vi "VdAnalogInput_Create.vi"(8 "Error In":errorcluster, 9 "VoltageRangeLow":dbl, 10 "VoltageRangeHigh":dbl, 11 "reference in":refnum<class "VdAnalogInput.lvclass">) -> (0 "Error Out":errorcluster, 3 "reference out":refnum<class "VdAnalogInput.lvclass">)   [LabVIEW 2020, in "VdAnalogInput.lvclass"]
uses:
  VdAnalogInput.lvclass
  VdAnalogInput.lvclass/VdAnalogInput.ctl
  VdInstrument_class/VdInstrument.lvclass
  C:/Projects/DesignPatterns/Factory1/VdInstrument_class/VdInstrument.lvclass
  C:/Projects/DesignPatterns/Factory1/VdAnalogInput_class/VdAnalogInput.lvclass
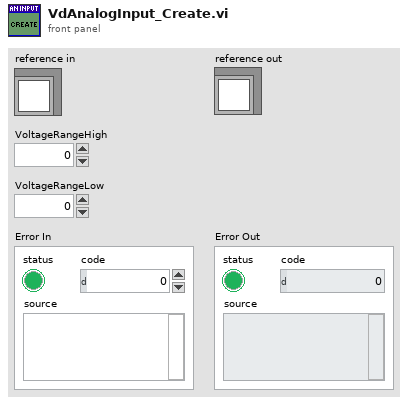
[diagram p1: front panel]
types:
  T1 = typedef "VdAnalogInput.lvclass/ObjectAttributes.ctl" = cluster{"LastReadValue":dbl, "VoltageRangeLow":dbl, "VoltageRangeHigh":dbl}
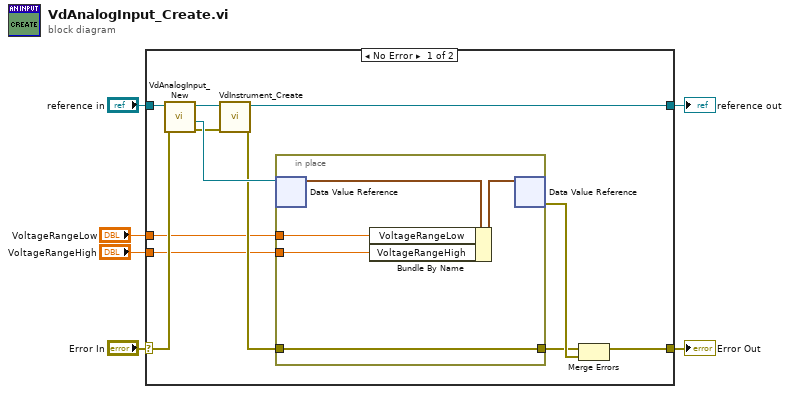
[diagram p0: block diagram]
diagram:
  n1 = case shown="No Error" "Error In" {
    selector: "Error In" -> [w14 w25]
    tunnel: [w12 w25] -> w5
    tunnel: "reference in" -> [w16 w24]
    tunnel: [w11 w24] -> w3
    tunnel: "VoltageRangeLow" -> [w8 _]
    tunnel: "VoltageRangeHigh" -> [w7 _]
    frame No Error {
      n2 = call "VdAnalogInput_New.vi"("error in (no error)"=w14, "reference in"=w16) -> ("error out"=w15:errorcluster, "DVRRefOut"=w18:refnum<data-value>, "reference out"=w17:refnum<class "VdAnalogInput.lvclass">)  [unwired: 6 in, 1 out]
      n3 = call "VdInstrument_Create.vi"("Error In"=w15, "reference in"=w17) -> ("Error Out"=w10:errorcluster, "reference out"=w11:refnum<class "VdAnalogInput.lvclass">)  [unwired: 8 in]
      n4 = in-place {
        in-place-border: w10 -> [w21]
        in-place-border: [w21] -> w9
        in-place-border: w8 -> [w20]
        in-place-border: w7 -> [w19]
        n5 = in-place-dvr #1(w18) -> (w22:T1)  [unwired: 1 out]
        n6 = Bundle By Name(cluster=w22, "VoltageRangeLow"=w20, "VoltageRangeHigh"=w19) -> (w23:T1)
        n7 = in-place-dvr #1(w23) -> (w13:errorcluster)  [unwired: 1 out]
      }
      n8 = Merge Errors(w9, w13) -> (w12:errorcluster)
    }
    frame Error {
    }
  }
  "Error Out" <- w5
  "reference out" <- w3
